vi "7th CMD Operations.vi"(8 "error in (no error)":errorcluster, 10 "Message In":refnum<class "Message.lvclass">, 11 "System Actor in":refnum<class "System Actor.lvclass">) -> (0 "error out":errorcluster, 2 "Stop":bool, 3 "System Actor out":refnum<class "System Actor.lvclass">)   [LabVIEW 2024, in "System Actor.lvclass"]
uses:
  System Actor.lvclass
  Message/Message.lvclass
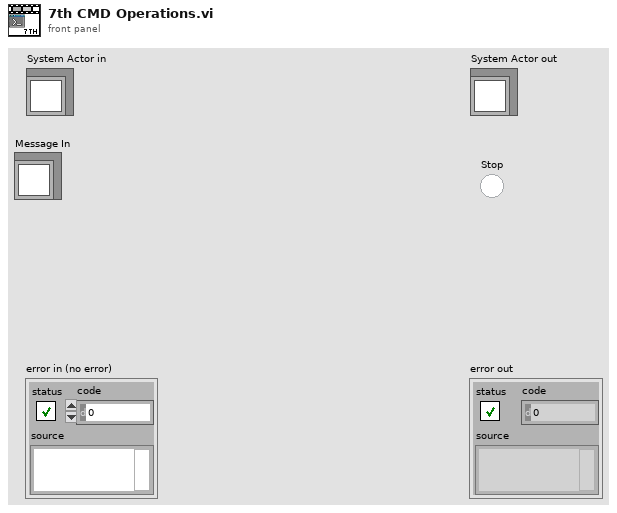
[diagram p1: front panel]
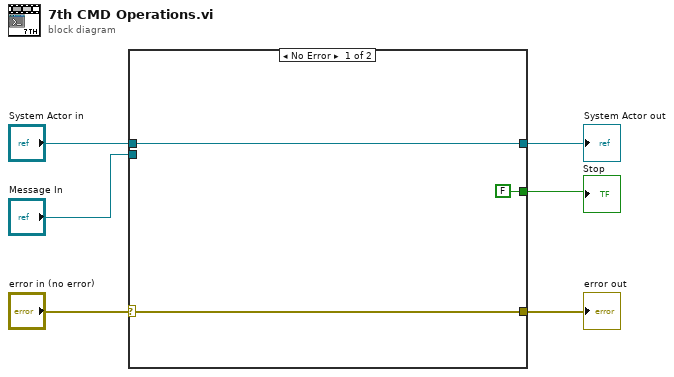
[diagram p0: block diagram]
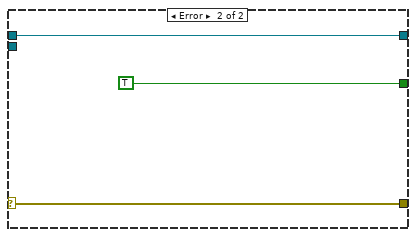
[diagram p2: hidden frame]
diagram:
  n1 = case shown="No Error" "error in (no error)" {
    selector: "error in (no error)" -> [w8 w12]
    tunnel: [w8 w12] -> w6
    tunnel: [w9 w11] -> w4
    tunnel: "System Actor in" -> [w9 w11]
    tunnel: [FALSE TRUE] -> w1
    tunnel: "Message In" -> [_ _]
    frame No Error {
    }
    frame Error {
    }
  }
  "error out" <- w6
  "System Actor out" <- w4
  "Stop" <- w1
